vi "WriteCWTravelLimit.vi"(8 "error in":errorcluster, 10 "CWTravelLimit":dbl, 11 "VISA resource name":refnum<visa-resource-name>) -> (0 "error out":errorcluster, 3 "VISA resource name out":refnum<visa-resource-name>)   [LabVIEW 2019, in "Mark 10 TSTM-DC.lvlib"]
uses:
  Mark 10 TSTM-DC.lvlib
  Mark 10 Event Monitor/Mark 10 Event Monitor.lvlib
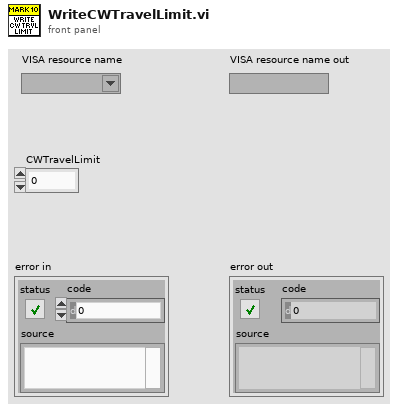
[diagram p1: front panel]
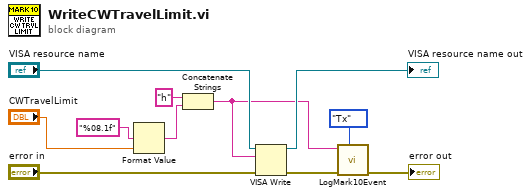
[diagram p0: block diagram]
diagram:
  n1 = Format Value(format string="%08.1f", value (0)="CWTravelLimit") -> (output string=w5:string)  [unwired: 1 in]
  n2 = Concatenate Strings("h" ("write buffer"), w5) -> (w2:string)
  n3 = VISA Write(VISA resource name="VISA resource name", write buffer=w2, error in (no error)="error in") -> (VISA resource name out=→"VISA resource name out":refnum<visa-resource-name>, error out=w9:errorcluster)  [unwired: 1 out]
  n4 = call "LogMark10Event.vi"("Type"=enum16{"Tx", "Rx"}."Tx", "Error In"=w9, "Event"=w2) -> ("Error Out"=→"error out":errorcluster)  [unwired: 8 in]
